vi "FgClass.vi"(7 "Set (F)":bool, 11 "Class In":refnum<class "ScopePluginsBase.lvclass">) -> (3 "Class Out":refnum<class "ScopePluginsBase.lvclass">)   [LabVIEW 2014, in "ScopeModule.lvlib"]
uses:
  ScopeModule.lvlib
  ScopePlugins/ScopePluginBaseClass/ScopePluginsBase.lvclass
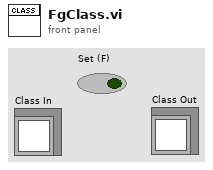
[diagram p1: front panel]
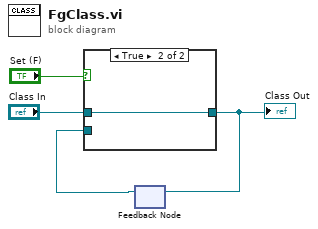
[diagram p0: block diagram]
diagram:
  n1 = feedback #1() -> (w1:refnum<class "ScopePluginsBase.lvclass">)  [unwired: 1 in]
  n2 = case shown="True" "Set (F)" {
    tunnel: "Class In" -> [_ w6]
    tunnel: [w5 w6] -> w2
    tunnel: w1 -> [w5 _]
    frame False {
    }
    frame True {
    }
  }
  "Class Out" <- w2
  n3 = feedback-in #1(w2) -> ()
